vi "SFOAE-Process Buffer.vi"(0 "DataProc In":T1, 7 "Buffer":dbl[](array[numeric]), 11 "error in (no error)":errorcluster) -> (4 "DataProc Out":T1, 8 "Nacq":i32, 14 "Finished":bool, 15 "error out":errorcluster)   [LabVIEW 2020]
uses:
  Typedefs/SFOAE-Data Processing.ctl
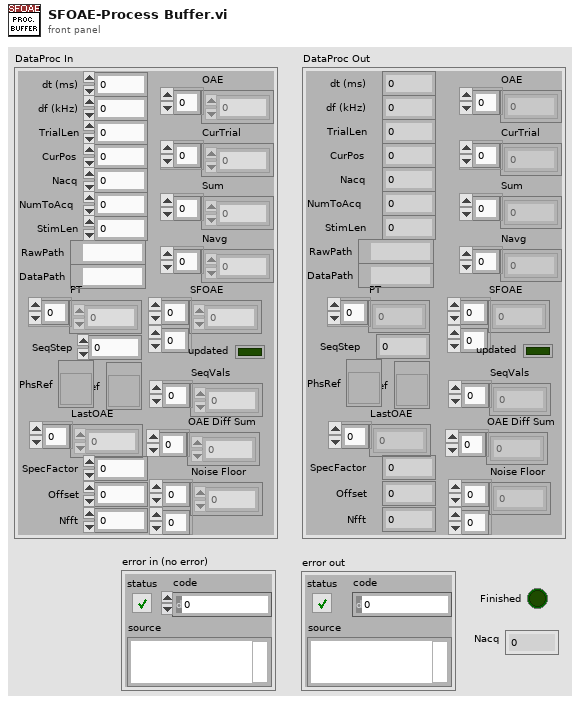
[diagram p1: front panel]
types:
  T1 = typedef "SFOAE-Data Processing.ctl" = cluster{"dt (ms)":dbl, "TrialLen":i32, "PT":cdb[], "CurPos":i32, "Sum":dbl[], "Navg":dbl[], "Nacq":i32, "RawPath":path, "DataPath":path, "NumToAcq":i32, "OAE":dbl[], "CurTrial":dbl[], "StimLen":i32, "SFOAE":cdb[][], "SeqStep":i32, "updated":bool, "SeqVals":dbl[], "df (kHz)":dbl, "MagRef":refnum<vi>, "LastOAE":dbl[], "OAE Diff Sum":dbl[], "Noise Floor":cdb[][], "SpecFactor":dbl, "Offset":i32, "Nfft":i32, "PhsRef":refnum<vi>}
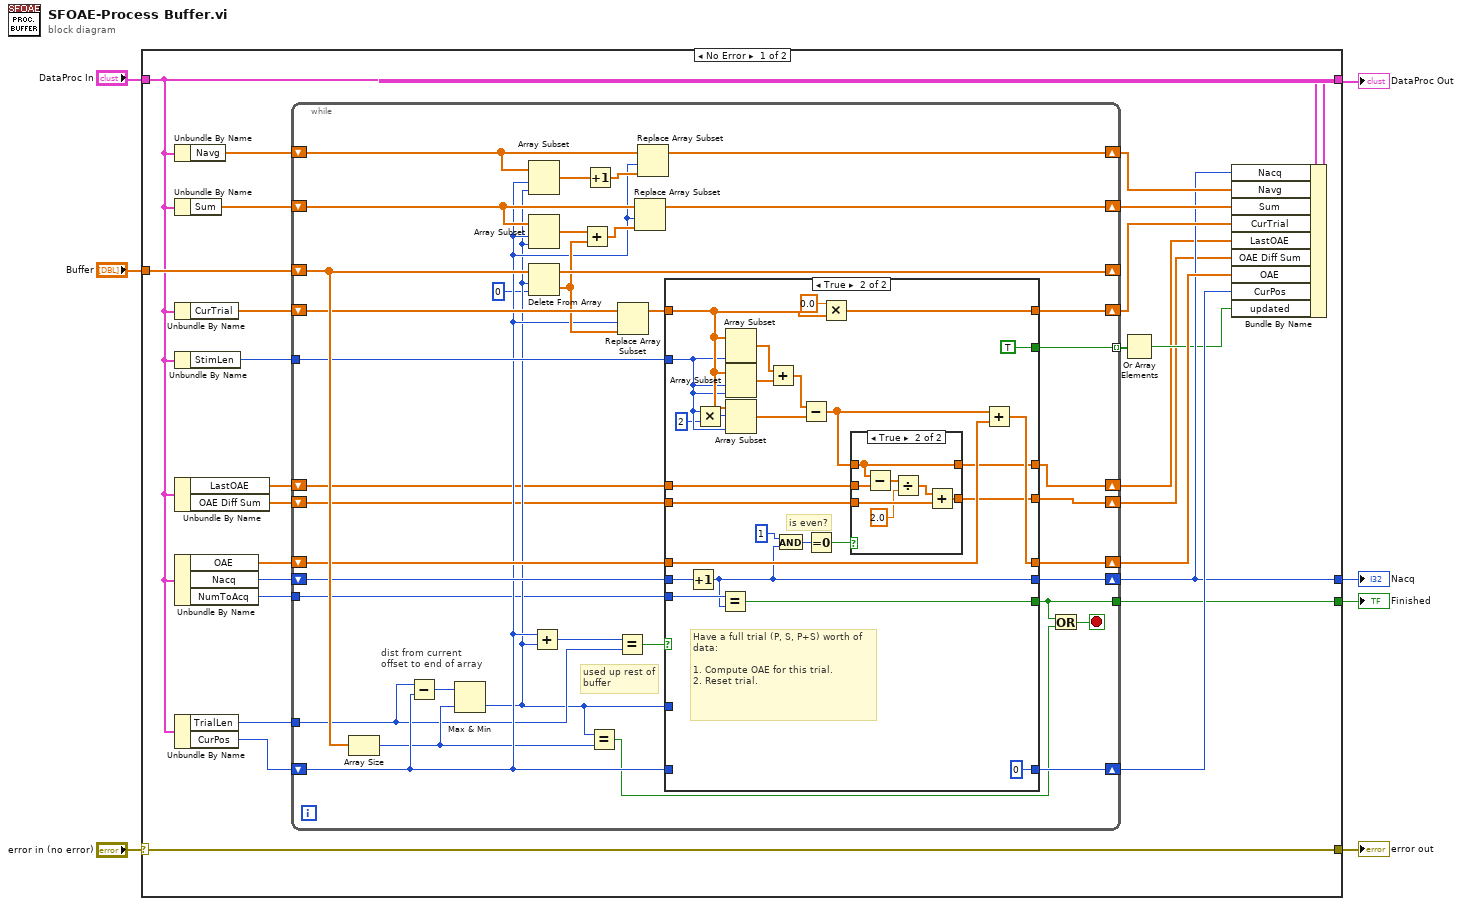
[diagram p0: block diagram]
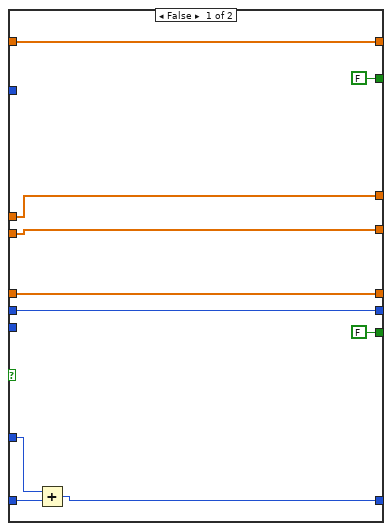
[diagram p2: hidden frame]
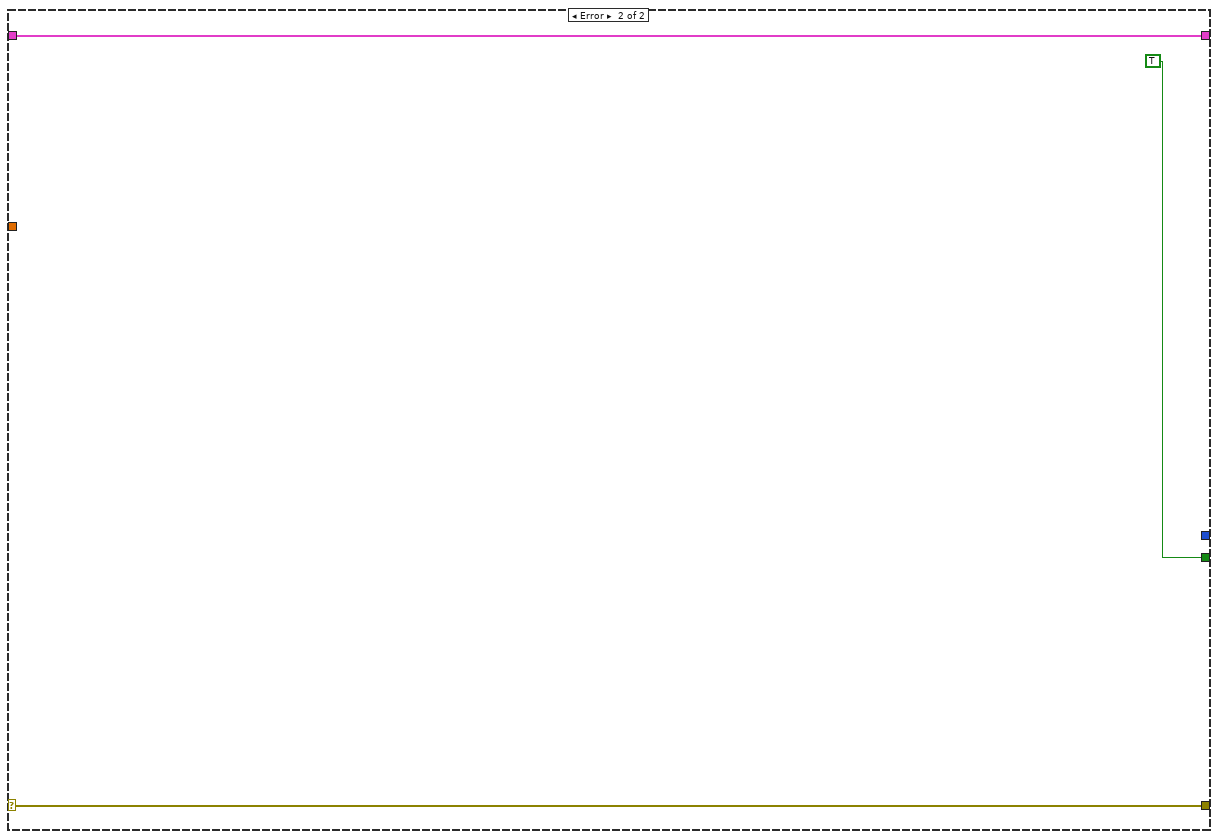
[diagram p4: hidden frame]
diagram:
  n1 = case shown="No Error" "error in (no error)" {
    selector: "error in (no error)" -> [w33 w117]
    tunnel: "DataProc In" -> [w12 w118]
    tunnel: [w27 w118] -> w4
    tunnel: [w33 w117] -> w6
    tunnel: "Buffer" -> [w30 _]
    tunnel: [w17 _] -> w2
    tunnel: [w15 TRUE] -> w1
    frame No Error {
      n2 = Unbundle By Name(w12) -> ("Navg"=w29:dbl[])
      n3 = Unbundle By Name(w12) -> ("Sum"=w31:dbl[])
      n4 = Unbundle By Name(w12) -> ("CurTrial"=w23:dbl[])
      n5 = Unbundle By Name(w12) -> ("StimLen"=w21:i32)
      n6 = Unbundle By Name(w12) -> ("LastOAE"=w11:dbl[], "OAE Diff Sum"=w9:dbl[])
      n7 = Unbundle By Name(w12) -> ("OAE"=w20:dbl[], "Nacq"=w19:i32, "NumToAcq"=w16:i32)
      n8 = Unbundle By Name(w12) -> ("TrialLen"=w32:i32, "CurPos"=w28:i32)
      n9 = while {
        tunnel: w32 -> [w45]
        shift-right: [w61] -> w24
        shift-left: w29 -> [w62]
        shift-right: [w68] -> w26
        shift-left: w31 -> [w67]
        shift-right: [w60] -> _
        shift-left: w30 -> [w65]
        shift-right: [w59] -> w25
        shift-left: w28 -> [w49]
        shift-right: [w55] -> w22
        shift-left: w23 -> [w58]
        tunnel: w21 -> [w54]
        shift-right: [w52] -> w18
        shift-left: w20 -> [w53]
        shift-right: [w50] -> w17
        shift-left: w19 -> [w51]
        tunnel: w16 -> [w42]
        tunnel: [w39] -> w15
        tunnel: [w38] -> w14 mode=indexing
        shift-right: [w34] -> w8
        shift-left: w9 -> [w35]
        shift-right: [w36] -> w10
        shift-left: w11 -> [w37]
        stop <- w41 stop-if-true
        # "used up rest of buffer"
        # "dist from current offset to end of array"
        n10 = Array Size(array=w65) -> (size(s)=w46:i32)
        n11 = Subtract(x=w45, y=w49) -> (x-y=w70:i32)
        n12 = Max & Min(x=w70, y=w46) -> (min(x,y)=w44:i32)  [unwired: 1 out]
        n13 = Array Subset(array=w62, index=w49, length=w44) -> (w64:dbl[])
        n14 = Array Subset(array=w67, index=w49, length=w44) -> (w69:dbl[])
        n15 = Delete From Array(array=w65, length=w44, index=0) -> (deleted portion=w57:dbl[], array with subset deleted=w60:dbl[])
        n16 = Add(x=w49, y=w44) -> (x+y=w48:i32)
        n17 = Add(x=w69, y=w57) -> (x+y=w66:dbl[])
        n18 = Increment(x=w64) -> (x+1=w63:dbl[])
        n19 = Equal?(x=w44, y=w46) -> (x = y?=w40:bool)
        n20 = Equal?(x=w48, y=w45) -> (x = y?=w47:bool)
        n21 = Replace Array Subset(array=w58, new element=w57, index=w49) -> (w56:dbl[])
        n22 = Replace Array Subset(array=w67, new element=w66, index=w49) -> (w68:dbl[])
        n23 = Replace Array Subset(array=w62, new element=w63, index=w49) -> (w61:dbl[])
        n24 = case shown="True" w47 {
          tunnel: w49 -> [w77 _]
          tunnel: [w75 0] -> w59
          tunnel: w56 -> [w80 w104]
          tunnel: [w80 w106] -> w55
          tunnel: w54 -> [_ w103]
          tunnel: w53 -> [w79 w97]
          tunnel: [w79 w96] -> w52
          tunnel: w51 -> [w78 w85]
          tunnel: [w78 w83] -> w50
          tunnel: w44 -> [w76 _]
          tunnel: w42 -> [_ w94]
          tunnel: [FALSE w93] -> w39
          tunnel: [FALSE TRUE] -> w38
          tunnel: w37 -> [w72 w91]
          tunnel: [w72 w89] -> w36
          tunnel: w35 -> [w71 w88]
          tunnel: [w71 w87] -> w34
          frame False {
            n25 = Add(x=w76, y=w77) -> (x+y=w75:i32)
          }
          frame True {
            # "is even?"
            # "Have a full trial (P, S, P+S) worth of data:\n\n1. Compute OAE for this trial.\n2. Reset trial."
            n26 = Increment(x=w85) -> (x+1=w83:i32)
            n27 = Multiply(x=w103, y=2) -> (x*y=w102:i32)
            n28 = Equal?(x=w94, y=w83) -> (x = y?=w93:bool)
            n29 = Array Subset(array=w104, length=w103) -> (w90:dbl[])  [unwired: 1 in]
            n30 = Array Subset(array=w104, index=w103, length=w103) -> (w100:dbl[])
            n31 = Array Subset(array=w104, index=w102, length=w103) -> (w98:dbl[])
            n32 = Add(x=w90, y=w100) -> (x+y=w99:dbl[])
            n33 = And(x=1, y=w83) -> (x .and. y?=w82:i32)
            n34 = Subtract(x=w99, y=w98) -> (x-y=w86:dbl[])
            n35 = Equal To 0?(x=w82) -> (x = 0?=w81:bool)
            n36 = Multiply(x=0.0 ("Numeric"), y=w104) -> (x*y=w106:dbl[])
            n37 = case shown="True" w81 {
              tunnel: w91 -> [_ w115]
              tunnel: w86 -> [w108 w113]
              tunnel: [w108 w113] -> w89
              tunnel: w88 -> [w107 w114]
              tunnel: [w107 w112] -> w87
              frame False {
              }
              frame True {
                n38 = Subtract(x=w113, y=w115) -> (x-y=w111:dbl[])
                n39 = Divide(x=w111, y=2.0) -> (x/y=w110:dbl[])
                n40 = Add(x=w110, y=w114) -> (x+y=w112:dbl[])
              }
            }
            n41 = Add(x=w86, y=w97) -> (x+y=w96:dbl[])
          }
        }
        n42 = Or(x=w39, y=w40) -> (x .or. y?=w41:bool)
      }
      n43 = Or Array Elements(Boolean array=w14) -> (logical OR=w13:bool)
      n44 = Bundle By Name(cluster=w12, "Nacq"=w17, "Navg"=w24, "Sum"=w26, "CurTrial"=w22, "LastOAE"=w10, "OAE Diff Sum"=w8, "OAE"=w18, "CurPos"=w25, "updated"=w13) -> (w27:T1)
    }
    frame Error {
    }
  }
  "error out" <- w6
  "DataProc Out" <- w4
  "Nacq" <- w2
  "Finished" <- w1
